vi "Test.vi"() -> ()   [LabVIEW 2020]
uses:
  XControl/Step Control/Step.xctl
panel:
  out "Read Process":u16[](array[ring])
  out "Scan Process":T1(array[cluster])
  in  "Update Read Instrument":string[](array[string])=["R0", "R1", "R2"]
  in  "Update Scan Instrument":string[](array[string])=["S0", "S1", "S2"]
  out "Step Set 2":T2(array[cluster])=[{"Wait(s)"=0.0, "Interplate Method"=0, "Read Process"=[], "Scan Process"=[{"Scan Instrument"=0, "Linear/Log"=FALSE, "Period/Number"=FALSE, "Balance Time(s)"=5.0, "Scan Parameter"=[]}], "Step Information"={"Step Name"="", "Step Description"=""}}] {"Interplate Method" items=["Recursion", "Sequence", "Merge"]}
  in  "Step":T2(xcontrol)=[{"Wait(s)"=0.0, "Interplate Method"=0, "Read Process"=[], "Scan Process"=[{"Scan Instrument"=0, "Linear/Log"=FALSE, "Period/Number"=FALSE, "Balance Time(s)"=5.0, "Scan Parameter"=[]}], "Step Information"={"Step Name"="", "Step Description"=""}}]
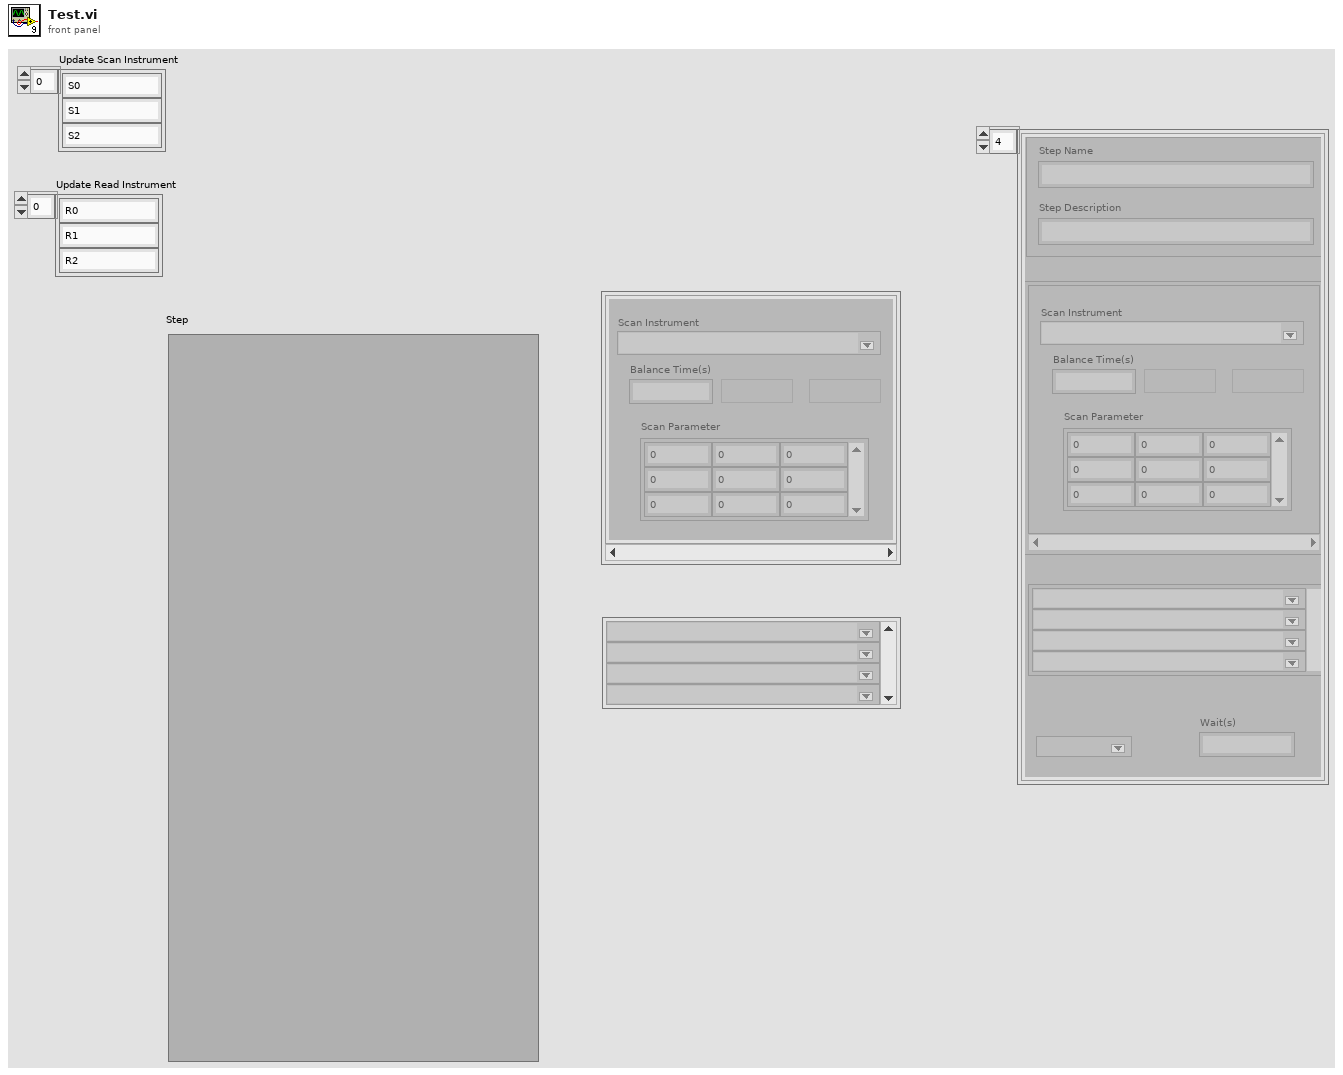
[diagram p1: front panel]
types:
  T1 = cluster{"Scan Instrument":u16, "Linear/Log":bool, "Period/Number":bool, "Balance Time(s)":dbl, "Scan Parameter":dbl[][]}[]
  T2 = cluster{"Wait(s)":dbl, "Interplate Method":u16, "Read Process":u16[], "Scan Process":cluster{"Scan Instrument":u16, "Linear/Log":bool, "Period/Number":bool, "Balance Time(s)":dbl, "Scan Parameter":dbl[][]}[], "Step Information":cluster{"Step Name":string, "Step Description":string}}[]
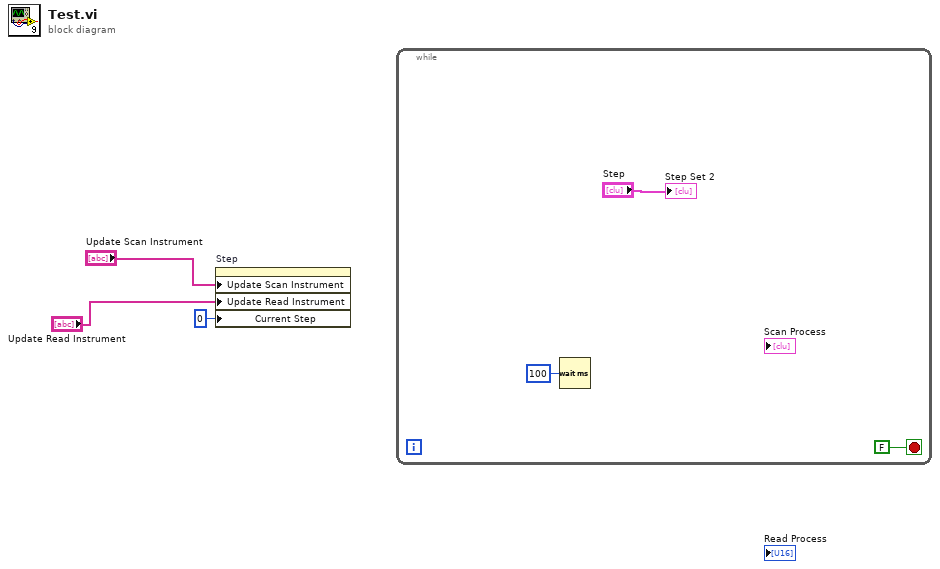
[diagram p0: block diagram]
diagram:
  n1 = property on="Step" class="Step (strict)"("Update Scan Instrument"="Update Scan Instrument", "Update Read Instrument"="Update Read Instrument", "Current Step"=0) -> ()  [unwired: 2 in, 2 out]
  n2 = while {
    stop <- FALSE stop-if-true
    n3 = Wait (ms)(milliseconds to wait=u32 100) -> ()  [unwired: 1 out]
    "Step Set 2" <- "Step"
  }
